vi "Check Limits.vi"(1 "Max Value":i16, 2 "Input":i16) -> (0 "Output":i16)   [LabVIEW 2011, in "OfflineTracker.lvlib"]
uses:
  OfflineTracker.lvlib
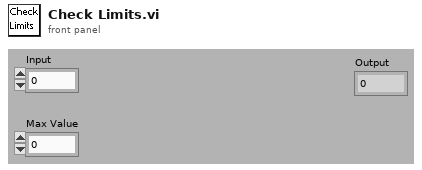
[diagram p1: front panel]
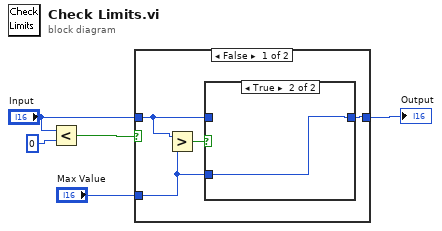
[diagram p0: block diagram]
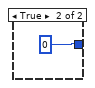
[diagram p3: hidden frame]
diagram:
  n1 = Less?(x="Input", y=i16 0) -> (x < y?=w3:bool)
  n2 = case shown="False" w3 {
    tunnel: [w9 0] -> w2
    tunnel: "Input" -> [w7 _]
    tunnel: "Max Value" -> [w6 _]
    frame False {
      n3 = Greater?(x=w7, y=w6) -> (0:w8:bool)
      n4 = case shown="True" w8 {
        tunnel: w7 -> [w10 _]
        tunnel: [w10 w11] -> w9
        tunnel: w6 -> [_ w11]
        frame False {
        }
        frame True {
        }
      }
    }
    frame True {
    }
  }
  "Output" <- w2
